vi "wa32 WaitNamedPipeA.vi"(8 "error in":errorcluster, 10 "timeout [ms]":u32=50, 11 "pipe name":string) -> (0 "error out":errorcluster)   [LabVIEW 2020, in "GOLPI library.lvlib"]
doc: "WinAPI WaitNamedPipeA() wrapper."
uses:
  <vilib>/Utility/error.llb/Error Cluster From Error Code.vi
  <vilib>/ErrorRing/Error Ring.xnode
  GOLPI library.lvlib
  kernel32.dll
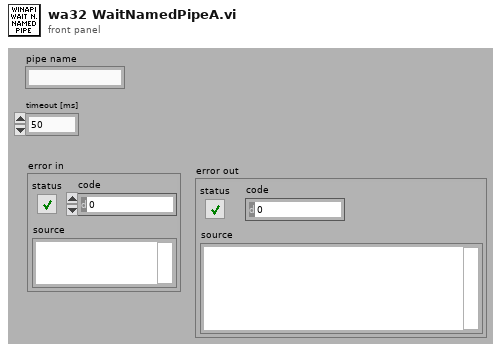
[diagram p1: front panel]
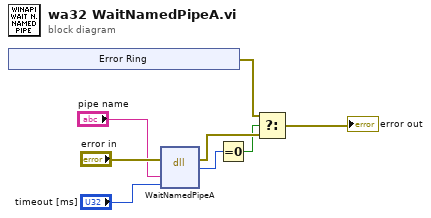
[diagram p0: block diagram]
diagram:
  n1 = xnode "Error Ring"() -> ("error out"=w5:errorcluster)
  n2 = dll-call lib="kernel32.dll" fn="WaitNamedPipeA"(error in="error in", "name"="pipe name", "timeout"="timeout [ms]") -> (error out=w7:errorcluster, "errout"=w4:i32)  [unwired: 4 in, 1 out]
  n3 = Equal To 0?(x=w4) -> (x = 0?=w3:bool)
  n4 = Select(t=w5, s=w3, f=w7) -> (s? t:f=→"error out":errorcluster)
